vi "Test 5.vi"() -> ()   [LabVIEW 2019]
panel:
  out "输出数组":i32[](array[numeric])
  out "元素":i32
  in  "索引":i32
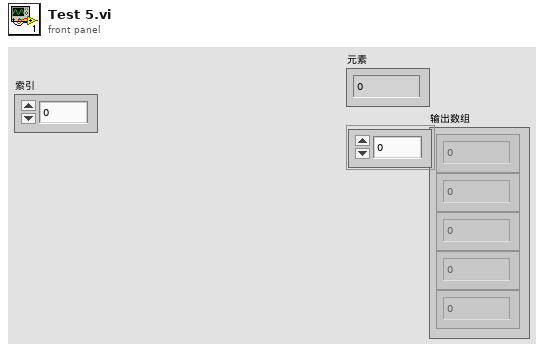
[diagram p1: front panel]
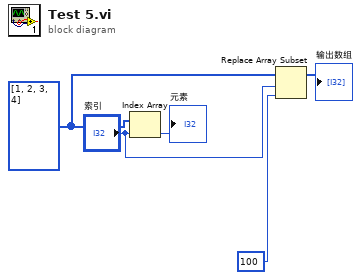
[diagram p0: block diagram]
diagram:
  w4 = i32[] [1, 2, 3, 4]
  n1 = Index Array(array=w4, index="索引") -> (element=→"元素":i32)
  n2 = Replace Array Subset(array=w4, new element=100 ("新元素/子数组"), index="索引") -> (→"输出数组":i32[])
